vi "ErrorHandling_Range_Set.vi"(8 "error in (no error)":errorcluster, 10 "Indices Set (for single index set upper value to -1)":cluster{"Lower value":i16, "Upper value":i16}[](array[cluster]), 11 "OXY_SCPI Reseource In":refnum<visa-resource-name>) -> (0 "error out":errorcluster, 1 "communication_data":T1, 3 "OXY_SCPI Reseource Out":refnum<visa-resource-name>)   [LabVIEW 2018, in "OXYGEN.lvlib"]
doc: "Add a range of error codes to be queued in the Error Queue"
uses:
  OXYGEN.lvlib
  TypeDefs/Cluster_RawCommData.ctl
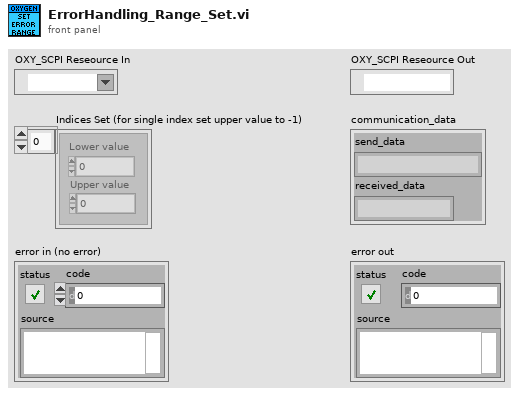
[diagram p1: front panel]
types:
  T1 = typedef "OXYGEN.lvlib/Cluster_RawCommData.ctl" = cluster{"send_data":string, "received_data":string}
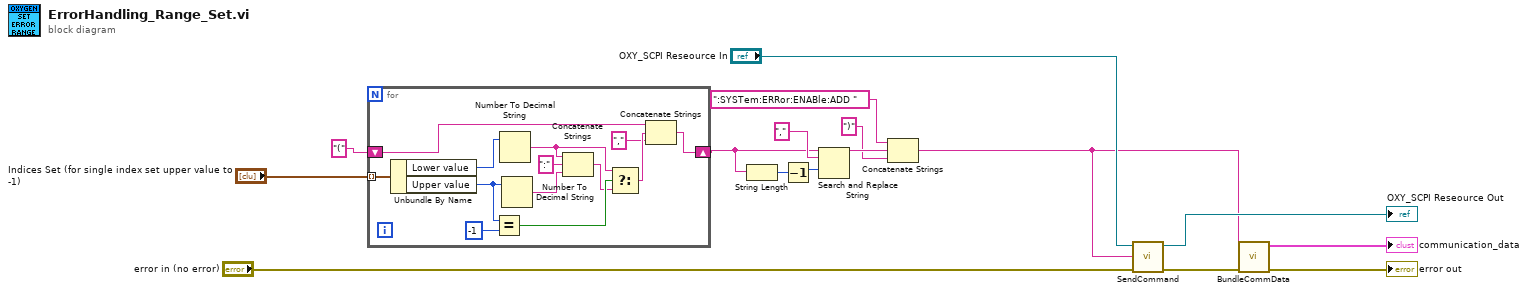
[diagram p0: block diagram]
diagram:
  n1 = for {
    tunnel: "Indices Set (for single index set upper value to -1)" -> [w29] mode=indexing
    shift-right: [w20] -> w5
    shift-left: "(" ("string") -> [w23]
    n2 = Unbundle By Name(w29) -> ("Lower value"=w28:i16, "Upper value"=w17:i16)
    n3 = Equal?(x=w17, y=i16 -1) -> (x = y?=w24:bool)
    n4 = Number To Decimal String(number=w28) -> (decimal integer string=w18:string)  [unwired: 1 in]
    n5 = Number To Decimal String(number=w17) -> (decimal integer string=w25:string)  [unwired: 1 in]
    n6 = Concatenate Strings(w18, ":" ("string"), w25) -> (w19:string)
    n7 = Select(t=w18, s=w24, f=w19) -> (s? t:f=w22:string)
    n8 = Concatenate Strings(w23, w22, "," ("string")) -> (w20:string)
  }
  n9 = String Length(string=w5) -> (length=w6:i32)
  n10 = Decrement(x=w6) -> (x-1=w8:i32)
  n11 = Search and Replace String(input string=w5, search string=",", offset=w8) -> (result string=w4:string)  [unwired: 5 in, 3 out]
  n12 = Concatenate Strings(":SYSTem:ERRor:ENABle:ADD " ("t"), w4, ")" ("string")) -> (w1:string)
  n13 = call "SendCommand.vi"("error in (no error)"="error in (no error)", "String to Send"=w1, "OXY_SCPI Reseource In"="OXY_SCPI Reseource In") -> ("error out"=w12:errorcluster, "OXY_SCPI Reseource Out"=→"OXY_SCPI Reseource Out":refnum<visa-resource-name>)  [unwired: 7 in]
  n14 = call "BundleCommData.vi"("error in (no error)"=w12, "send_data"=w1) -> ("error out"=→"error out":errorcluster, "communication_data"=→"communication_data":T1)  [unwired: 8 in]
